vi "Close - NI.vi"(8 "error in (no error)":errorcluster, 11 "instrument handle":refnum<k15>) -> (0 "error out":errorcluster)   [LabVIEW 2020]
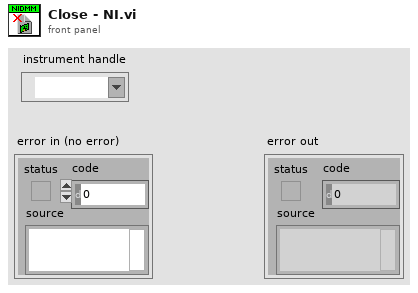
[diagram p1: front panel]
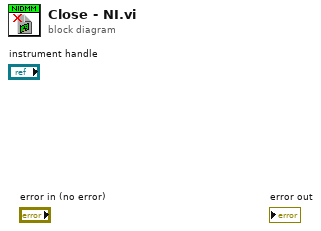
[diagram p0: block diagram]
diagram:
